vi "Config Write Part Type.vi"   [LabVIEW 2018]
uses:
  <vilib>/Utility/config.llb/Write Key (String).vi
  <vilib>/Utility/config.llb/NI_LVConfig.lvlib
types:
  T1 = typedef "NI_LVConfig.lvlib/Config Data RefNum.ctl" = refnum<k1>
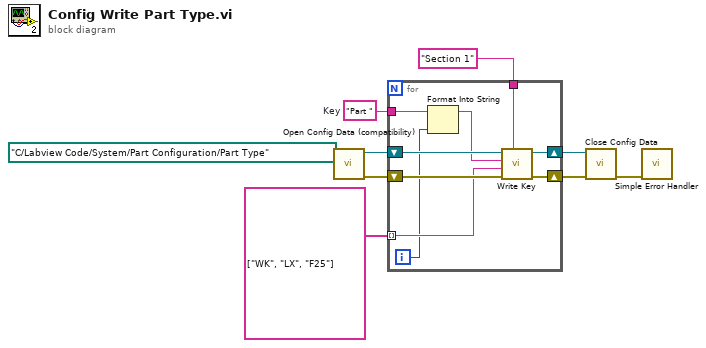
[diagram p0: block diagram]
diagram:
  w9 = "Part "  # Key
  n1 = call <vilib>:"Open Config Data (compatibility).vi"("configuration file path"=path "C:/Labview Code/System/Part Configuration/Part Type") -> ("error out"=w6:errorcluster, "refnum"=w7:T1)  [unwired: 8 in, 1 out]
  n2 = for {
    tunnel: w9 -> [w11]
    tunnel: "Section 1" -> [w14]
    shift-right: [w16] -> w4
    shift-left: w7 -> [w18]
    shift-right: [w15] -> w3
    shift-left: w6 -> [w17]
    tunnel: string[] ["WK", "LX", "F25"] -> [w13] mode=indexing
    i -> [w12]
    n3 = Format Into String(initial string=w11, w12) -> (resulting string=w10:string)  [unwired: 2 in, 1 out]
    n4 = call-poly <vilib>:"Write Key.vi"("section"=w14, "error in (no error)"=w17, "value"=w13, "key"=w10, "refnum"=w18) -> ("error out"=w15:errorcluster, "refnum out"=w16:T1)  [unwired: 4 in, 1 out]
  }
  n5 = call <vilib>:"Close Config Data.vi"("error in (no error)"=w3, "refnum"=w4) -> ("error out"=w8:errorcluster)  [unwired: 8 in, 1 out]
  n6 = call <vilib>:"Simple Error Handler.vi"("error in (no error)"=w8) -> ()  [unwired: 4 in, 5 out]
